vi "lcr tune mod.vi"() -> ()   [LabVIEW 2018]
uses:
  <vilib>/Analysis/NI_AALBase.lvlib
  <vilib>/Analysis/NI_AAL_SigProc.lvlib
  a6659894-6288-4190-a3c4-d24321de4737.vi
  <vilib>/DAQmx/write.llb/DAQmx Write (Analog DBL 1Chan 1Samp).vi
  <vilib>/DAQmx/create/channels.llb/DAQmx Create Channel (AO-Voltage-Basic).vi
  <vilib>/DAQmx/create/channels.llb/DAQmx Create Channel (AI-Voltage-Basic).vi
  2a3dda8a-b8aa-4613-8376-8d8c81e86704.vi
  <vilib>/Analysis/baseanly.llb/Mean (DBL).vi
  <vilib>/DAQmx/read.llb/DAQmx Read (Analog DBL 1Chan 1Samp).vi
panel:
  in  "stop":bool
  out "XY Graph 2":cluster{dbl[], dbl[]}(graph)={[0.0, 0.04950495049504951, 0.09900990099009901, 0.14851485148514854, 0.19801980198019803, 0.24752475247524752, 0.29702970297029707, 0.34653465346534656, 0.39603960396039606, 0.44554455445544555, 0.49504950495049505, 0.5445544554455446, 0.5940594059405941, 0.6435643564356436, 0.6930693069306931, 0.7425742574257426, 0.7920792079207921, 0.8415841584158417, 0.8910891089108911, 0.9405940594059407, 0.9900990099009901, 1.0396039603960396, 1.0891089108910892, 1.1386138613861387, 1.1881188118811883, 1.2376237623762376, 1.2871287128712872, 1.3366336633663367, 1.3861386138613863, 1.4356435643564358, 1.4851485148514851, 1.5346534653465347, 1.5841584158415842, 1.6336633663366338, 1.6831683168316833, 1.7326732673267327, 1.7821782178217822, 1.8316831683168318, 1.8811881188118813, 1.9306930693069309, 1.9801980198019802, 2.0297029702970297, 2.0792079207920793, 2.128712871287129, 2.1782178217821784, 2.227722772277228, 2.2772277227722775, 2.326732673267327, 2.3762376237623766, 2.4257425742574257, 2.4752475247524752, 2.5247524752475248, 2.5742574257425743, 2.623762376237624, 2.6732673267326734, 2.722772277227723, 2.7722772277227725, 2.821782178217822, 2.8712871287128716, 2.9207920792079207, 2.9702970297029703, 3.01980198019802, 3.0693069306930694, 3.118811881188119, 3.1683168316831685, 3.217821782178218, 3.2673267326732676, 3.316831683168317, 3.3663366336633667, 3.415841584158416, 3.4653465346534653, 3.514851485148515, 3.5643564356435644, 3.613861386138614, 3.6633663366336635, 3.712871287128713, 3.7623762376237626, 3.811881188118812, 3.8613861386138617, 3.9108910891089113, 3.9603960396039604, 4.00990099009901, 4.0594059405940595, 4.108910891089109, 4.158415841584159, 4.207920792079208, 4.257425742574258, 4.306930693069307, 4.356435643564357, 4.405940594059406, 4.455445544554456, 4.504950495049505, 4.554455445544555, 4.6039603960396045, 4.653465346534654, 4.702970297029704, 4.752475247524753, 4.801980198019802, 4.851485148514851, 4.900990099009901, 4.9504950495049505, 5.0], [3.6269698987299557, 3.6364573449364106, 3.6329899671345474, 3.6282543529705342, 3.629159309363951, 3.6287473758170243, 3.6300350736155056, 3.629924792216151, 3.6336451685832807, 3.63122870790565, 3.6250464609928272, 3.6300902143756275, 3.637209853485964, 3.6333467600149016, 3.630025342964688, 3.6329121214483715, 3.6278326887176044, 3.6270445008971244, 3.6230613953263267, 3.630712980049897, 3.6313000664504536, 3.6289971308177837, 3.6302329315360238, 3.6329153650017383, 3.6294609615211413, 3.63600000136827, 3.627411024462163, 3.6284100444363565, 3.6275861772915365, 3.6304729557761015, 3.629473935783759, 3.63204933151817, 3.6254162280427176, 3.627398050221512, 3.6295193457817647, 3.6331878249951624, 3.6319941907248854, 3.6278034965744808, 3.6220396703232898, 3.6262952359408596, 3.6273688580229018, 3.6348777256768994, 3.6264476837299795, 3.633719770708133, 3.6360843342001994, 3.6295290764943395, 3.6302459057692227, 3.6275504979969018, 3.6291366044222984, 3.632672097159256, 3.6235057645788302, 3.6296361143819986, 3.6328342757014656, 3.6316990257371065, 3.62449829739106, 3.629097681502316, 3.624031223133673, 3.6252702673373305, 3.6278229579737187, 3.6336192199758655, 3.6273623709287937, 3.621828838189813, 3.631844986473933, 3.625150255217819, 3.625172960190463, 3.6291917451084803, 3.6294479872235597, 3.619243711878944, 3.6345630992469626, 3.6295615122275064, 3.6293896029595634, 3.6309984143274994, 3.6328083271841956, 3.6245664123692127, 3.6280954180164486, 3.627754843002688, 3.6386662170654303, 3.62156935249656, 3.6349231357495135, 3.637310404233228, 3.6250724094892646, 3.6337684242639474, 3.638114809914663, 3.625224857360931, 3.6308427229410554, 3.637796939897928, 3.6351177500173657, 3.6332105299869375, 3.632360714266952, 3.635607529201048, 3.6308200179121477, 3.634835559237383, 3.6350820706466345, 3.6253027030898712, 3.633823564980328, 3.623252765981493, 3.6300156121881697, 3.6215855703379147, 3.6359124249670454, 3.630398353613972, 3.6265287730372937, 3.6269212451486847]}
  in  "width":i32=3 min=3
  in  "threshold":dbl format="%0.2f"
  in  "sample length":i32=100
  in  "Step length (ms)":dbl
  in  "step size":dbl
  out "estimated polarization":dbl
  in  "background intensity":dbl
  in  "polarimeter angle":dbl
  in  "pressure factor":dbl
  out "min location":dbl
  out "min value":dbl
  out "max location":dbl
  out "max value":dbl
  out "average":dbl
  in  "laser tune voltage":dbl=3.79 min=0.0 max=4.0 step=0.01
  out "max value":dbl=3.6386662170654303
  out "min value":dbl=3.619243711878944
  out "Voltage at min":dbl=3.316831683168317
  out "Voltage at max":dbl=3.7623762376237626
  out "Current Voltage":dbl=5.0
  out "XY Graph":cluster{dbl[], dbl[]}(graph)={[0.0, 0.04950495049504951, 0.09900990099009901, 0.14851485148514854, 0.19801980198019803, 0.24752475247524752, 0.29702970297029707, 0.34653465346534656, 0.39603960396039606, 0.44554455445544555, 0.49504950495049505, 0.5445544554455446, 0.5940594059405941, 0.6435643564356436, 0.6930693069306931, 0.7425742574257426, 0.7920792079207921, 0.8415841584158417, 0.8910891089108911, 0.9405940594059407, 0.9900990099009901, 1.0396039603960396, 1.0891089108910892, 1.1386138613861387, 1.1881188118811883, 1.2376237623762376, 1.2871287128712872, 1.3366336633663367, 1.3861386138613863, 1.4356435643564358, 1.4851485148514851, 1.5346534653465347, 1.5841584158415842, 1.6336633663366338, 1.6831683168316833, 1.7326732673267327, 1.7821782178217822, 1.8316831683168318, 1.8811881188118813, 1.9306930693069309, 1.9801980198019802, 2.0297029702970297, 2.0792079207920793, 2.128712871287129, 2.1782178217821784, 2.227722772277228, 2.2772277227722775, 2.326732673267327, 2.3762376237623766, 2.4257425742574257, 2.4752475247524752, 2.5247524752475248, 2.5742574257425743, 2.623762376237624, 2.6732673267326734, 2.722772277227723, 2.7722772277227725, 2.821782178217822, 2.8712871287128716, 2.9207920792079207, 2.9702970297029703, 3.01980198019802, 3.0693069306930694, 3.118811881188119, 3.1683168316831685, 3.217821782178218, 3.2673267326732676, 3.316831683168317, 3.3663366336633667, 3.415841584158416, 3.4653465346534653, 3.514851485148515, 3.5643564356435644, 3.613861386138614, 3.6633663366336635, 3.712871287128713, 3.7623762376237626, 3.811881188118812, 3.8613861386138617, 3.9108910891089113, 3.9603960396039604, 4.00990099009901, 4.0594059405940595, 4.108910891089109, 4.158415841584159, 4.207920792079208, 4.257425742574258, 4.306930693069307, 4.356435643564357, 4.405940594059406, 4.455445544554456, 4.504950495049505, 4.554455445544555, 4.6039603960396045, 4.653465346534654, 4.702970297029704, 4.752475247524753, 4.801980198019802, 4.851485148514851, 4.900990099009901, 4.9504950495049505, 5.0], [3.6269698987299557, 3.6364573449364106, 3.6329899671345474, 3.6282543529705342, 3.629159309363951, 3.6287473758170243, 3.6300350736155056, 3.629924792216151, 3.6336451685832807, 3.63122870790565, 3.6250464609928272, 3.6300902143756275, 3.637209853485964, 3.6333467600149016, 3.630025342964688, 3.6329121214483715, 3.6278326887176044, 3.6270445008971244, 3.6230613953263267, 3.630712980049897, 3.6313000664504536, 3.6289971308177837, 3.6302329315360238, 3.6329153650017383, 3.6294609615211413, 3.63600000136827, 3.627411024462163, 3.6284100444363565, 3.6275861772915365, 3.6304729557761015, 3.629473935783759, 3.63204933151817, 3.6254162280427176, 3.627398050221512, 3.6295193457817647, 3.6331878249951624, 3.6319941907248854, 3.6278034965744808, 3.6220396703232898, 3.6262952359408596, 3.6273688580229018, 3.6348777256768994, 3.6264476837299795, 3.633719770708133, 3.6360843342001994, 3.6295290764943395, 3.6302459057692227, 3.6275504979969018, 3.6291366044222984, 3.632672097159256, 3.6235057645788302, 3.6296361143819986, 3.6328342757014656, 3.6316990257371065, 3.62449829739106, 3.629097681502316, 3.624031223133673, 3.6252702673373305, 3.6278229579737187, 3.6336192199758655, 3.6273623709287937, 3.621828838189813, 3.631844986473933, 3.625150255217819, 3.625172960190463, 3.6291917451084803, 3.6294479872235597, 3.619243711878944, 3.6345630992469626, 3.6295615122275064, 3.6293896029595634, 3.6309984143274994, 3.6328083271841956, 3.6245664123692127, 3.6280954180164486, 3.627754843002688, 3.6386662170654303, 3.62156935249656, 3.6349231357495135, 3.637310404233228, 3.6250724094892646, 3.6337684242639474, 3.638114809914663, 3.625224857360931, 3.6308427229410554, 3.637796939897928, 3.6351177500173657, 3.6332105299869375, 3.632360714266952, 3.635607529201048, 3.6308200179121477, 3.634835559237383, 3.6350820706466345, 3.6253027030898712, 3.633823564980328, 3.623252765981493, 3.6300156121881697, 3.6215855703379147, 3.6359124249670454, 3.630398353613972, 3.6265287730372937, 3.6269212451486847]}
  in  "End Voltage":dbl=5.0 min=0.0 max=25.0 step=0.001 format="%#.3f"
  in  "VISA resource name":refnum<visa-resource-name>="LCC25"
  in  "Start Voltage":dbl min=0.0 max=25.0 step=0.001 format="%#.3f"
  # "This VI sweeps the LCR driving voltage.   LCR slow axis should be aligned to roughly 45 degrees from the \ntransmission axis of the linear plarizer.  The max and min of graph represent citical values such as 1/4 wave,\n3/4 wave, etc.  The corresponding Voltages are then used fine tune the alignemnt and to make polarization\nmeasurements."
  # "X"
  # "Y"
  # "(ignore for background measurements)"
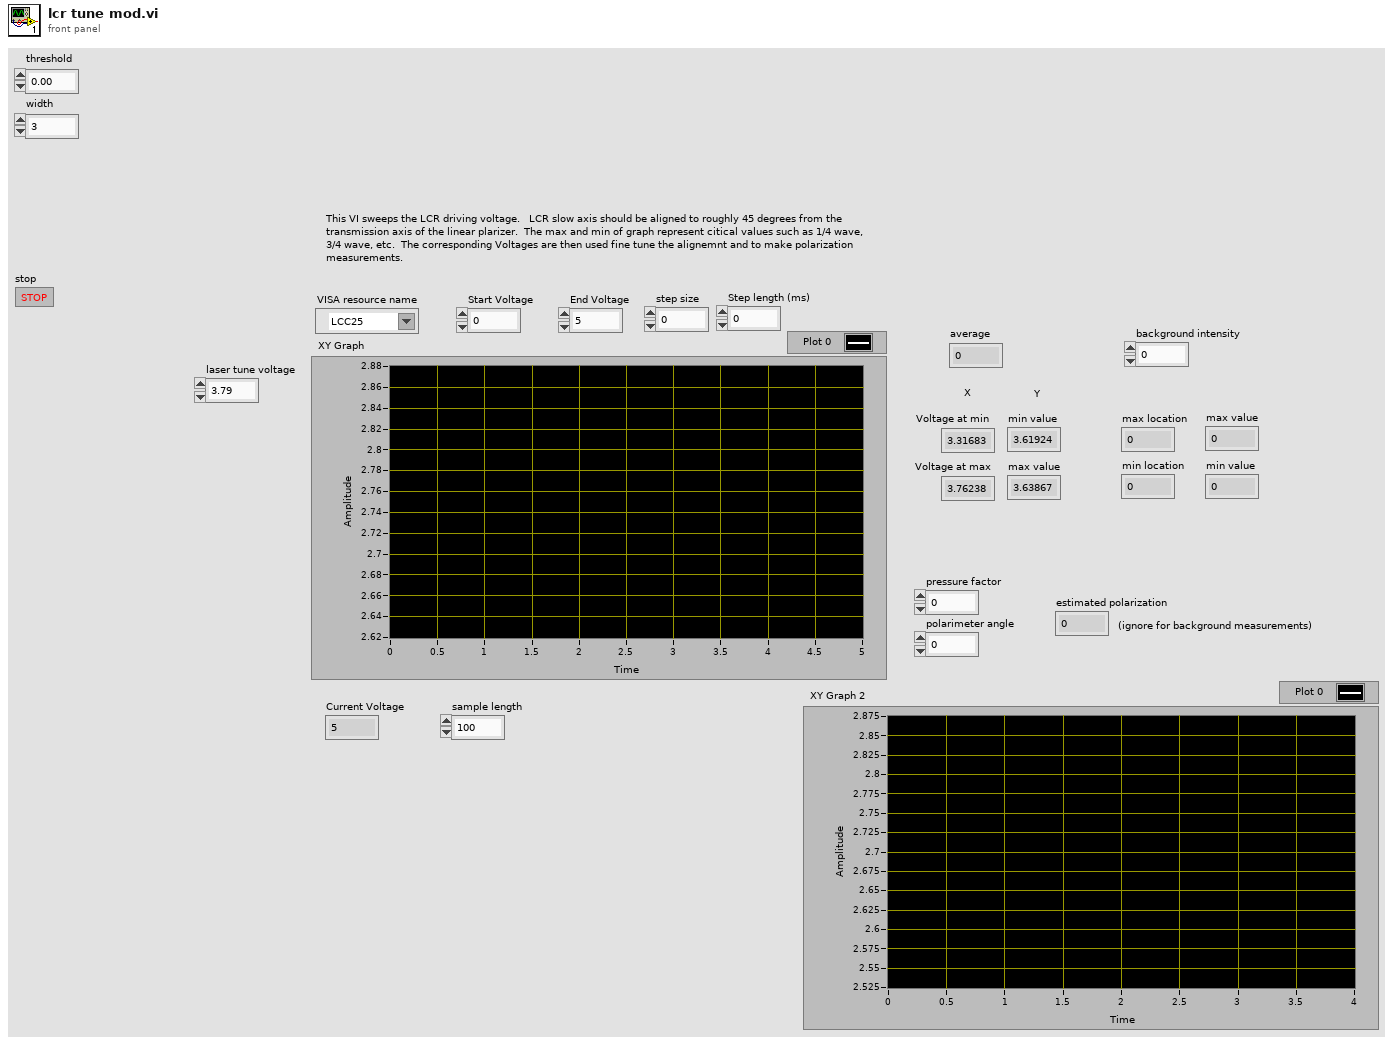
[diagram p1: front panel]
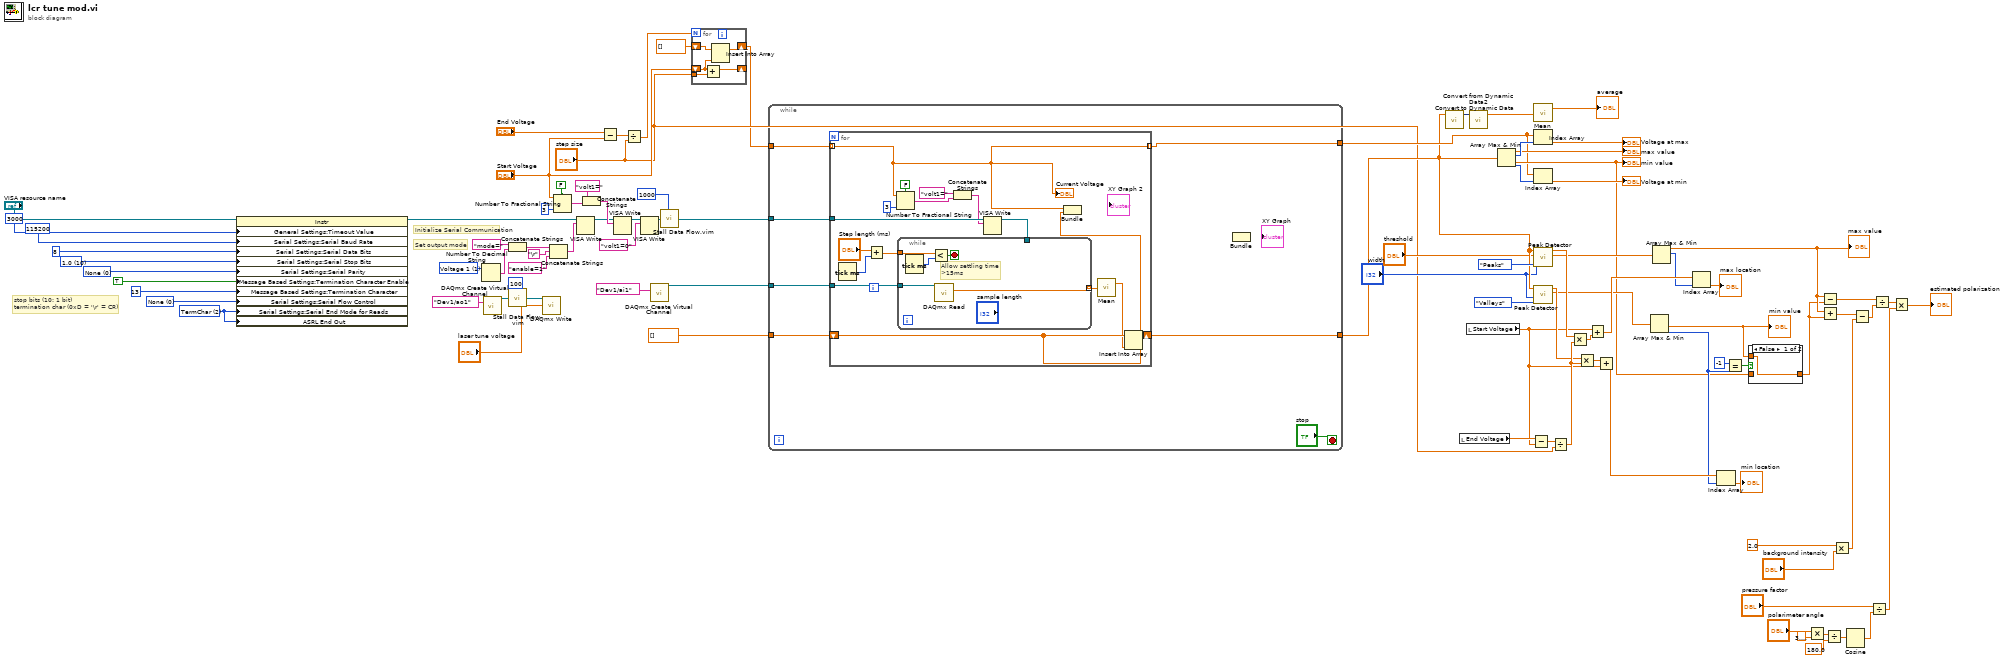
[diagram p0: block diagram]
diagram:
  w88 = u16 1 items=["Modulate", "Voltage 1", "Voltage 2"] ("Output Mode")
  w89 = u16 2 items=["None", "LastBit", "TermChar"] ("Serial Settings:Serial End Mode for Reads")
  w93 = u16 0 items=["None", "XON/XOFF", "RTS/CTS", "XON/XOFF & RTS/CTS", "DTR/DSR", "XON/XOFF & DTR/DSR"] ("flow control (0:none)")
  w91 = u16 0 items=["None", "Odd", "Even", "Mark", "Space"] ("Serial Settings:Parity")
  w95 = u16 10 items=["1.0"=10, "1.5"=15, "2.0"=20]
  # "stop bits (10: 1 bit)\ntermination char (0xD = '\\r' = CR)"
  # "Set output mode"
  # "Initialize Serial Communication"
  n1 = property class="Instr"(reference="VISA resource name", "General Settings:Timeout Value"=u32 3000 ("timeout (10sec)"), "Serial Settings:Serial Baud Rate"=u32 115200 ("baud rate (9600)115200"), "Serial Settings:Serial Data Bits"=u16 8 ("data bits (8)"), "Serial Settings:Serial Stop Bits"=w95, "Serial Settings:Serial Parity"=w91, "Message Based Settings:Termination Character Enable"=TRUE ("Enable Termination\nChar (T)"), "Message Based Settings:Termination Character"=u8 13, "Serial Settings:Serial Flow Control"=w93, "Serial Settings:Serial End Mode for Reads"=w89, "ASRL End Out"=w89) -> (reference out=w73:refnum<visa-resource-name>)  [unwired: 1 in, 1 out]
  n2 = Number To Decimal String(number=w88) -> (decimal integer string=w87:string)  [unwired: 1 in]
  n3 = call-poly <vilib>:"DAQmx Create Virtual Channel.vi"("physical channels"=tag "Dev1/ao1") -> ("task out"=w64:refnum<k21>)  [unwired: 13 in, 1 out]
  n4 = Concatenate Strings("mode=" ("string"), w87) -> (w75:string)
  n5 = call "Stall Data Flow.vim"("value in"=w64, "milliseconds to wait"=u32 100) -> ("value out"=w15:refnum<k21>)  [unwired: 1 out]
  n6 = call-poly <vilib>:"DAQmx Write.vi"("task/channels in"=w15, "data"="laser tune voltage") -> ()  [unwired: 11 in, 3 out]
  n7 = Concatenate Strings(w75, "\r", "enable=1" ("write buffer")) -> (w74:string)
  n8 = Number To Fractional String(use system decimal point (T)=FALSE, number="Start Voltage", precision (6)=i16 3) -> (F-format string=w69:string)  [unwired: 1 in]
  n9 = VISA Write(VISA resource name=w73, write buffer=w74) -> (VISA resource name out=w66:refnum<visa-resource-name>)  [unwired: 1 in, 2 out]
  n10 = Concatenate Strings("volt1=" ("string"), w69) -> (w67:string)
  n11 = Subtract(x="End Voltage", y="Start Voltage") -> (x-y=w84:dbl)
  n12 = VISA Write(VISA resource name=w66, write buffer=w67) -> (VISA resource name out=w29:refnum<visa-resource-name>)  [unwired: 1 in, 2 out]
  n13 = Divide(x=w84, y="step size") -> (x/y=w5:dbl)
  n14 = VISA Write(VISA resource name=w29, write buffer="volt1=0" ("string")) -> (VISA resource name out=w53:refnum<visa-resource-name>)  [unwired: 1 in, 2 out]
  n15 = call-poly <vilib>:"DAQmx Create Virtual Channel.vi"("physical channels"=tag "Dev1/ai1") -> ("task out"=w13:refnum<k21>)  [unwired: 13 in, 1 out]
  n16 = call "Stall Data Flow.vim"("value in"=w53, "milliseconds to wait"=u32 1000) -> ("value out"=w7:refnum<visa-resource-name>)  [unwired: 1 out]
  n17 = for {
    N: w5 -> [_]
    shift-right: [w100] -> w1
    shift-left: dbl[] [] -> [w101]
    tunnel: "step size" -> [w99]
    shift-right: [w98] -> _
    shift-left: "Start Voltage" -> [w97]
    n18 = Add(x=w97, y=w99) -> (x+y=w98:dbl)
    n19 = Insert Into Array(array=w101, new element=w97) -> (w100:dbl[])  [unwired: 1 in]
  }
  n20 = while {
    tunnel: [w108] -> w16
    tunnel: w13 -> [w107]
    tunnel: [w106] -> w11
    tunnel: dbl[] [] -> [w105]
    tunnel: w1 -> [w104]
    tunnel: w7 -> [w103]
    stop <- "stop" stop-if-true
    n21 = for {
      tunnel: w103 -> [w120]
      tunnel: w107 -> [w118]
      shift-right: [w113] -> w106
      shift-left: w105 -> [w112]
      tunnel: w104 -> [w109] mode=indexing
      tunnel: [w109] -> w108 mode=indexing
      n22 = Tick Count (ms)() -> (millisecond timer value=w117:u32)
      n23 = Add(x="Step length (ms)", y=w117) -> (x+y=w115:dbl)
      n24 = Number To Fractional String(use system decimal point (T)=FALSE, number=w109, precision (6)=i16 3) -> (F-format string=w122:string)  [unwired: 1 in]
      n25 = Concatenate Strings("volt1=" ("string"), w122) -> (w119:string)
      n26 = VISA Write(VISA resource name=w120, write buffer=w119) -> (VISA resource name out=w114:refnum<visa-resource-name>)  [unwired: 1 in, 2 out]
      n27 = while {
        tunnel: w118 -> [w129]
        tunnel: w115 -> [w128]
        tunnel: w114 -> [_]
        tunnel: [w125] -> w111 mode=indexing
        stop <- w126 stop-if-true
        # "Allow settling time\n>15ms"
        n28 = Tick Count (ms)() -> (millisecond timer value=w127:u32)
        n29 = Less?(x=w128, y=w127) -> (x < y?=w126:bool)
        n30 = call-poly <vilib>:"DAQmx Read.vi"("task/channels in"=w129) -> ("data"=w125:dbl)  [unwired: 12 in, 2 out]
      }
      n31 = Bundle(w109, w112) -> ()  [unwired: 1 in, 1 out]
      n32 = call-poly <vilib>:"Mean.vi"("X"=w111) -> ("mean"=w110:dbl)  [unwired: 1 out]
      n33 = Insert Into Array(array=w112, new element=w110) -> (w113:dbl[])  [unwired: 1 in]
      "Current Voltage" <- w109
    }
    n34 = Bundle() -> ()  [unwired: 3 in, 1 out]
  }
  n35 = call "Convert to Dynamic Data"("Array"=w11) -> ("Dynamic Data Type"=w27:dynamicdata)  [unwired: 3 in]
  n36 = local read "End Voltage"() -> (w62:dbl)
  n37 = local read "Start Voltage"() -> (w44:dbl)
  n38 = call "Convert from Dynamic Data2"("Dynamic Data Type"=w27) -> ("Array"=w52:dbl[])  [unwired: 3 in]
  n39 = Array Max & Min(array=w11) -> (max value=→"max value":dbl, max index (indices)=w81:i32, min value=w20:dbl, min index (indices)=w82:i32)
  "min value" <- w20
  n40 = Subtract(x=w62, y=w44) -> (x-y=w55:dbl)
  n41 = call-poly <vilib>:"Mean.vi"("X"=w52) -> ("mean"=→"average":dbl)  [unwired: 1 out]
  n42 = Index Array(array=w16, index=w81) -> (element=→"Voltage at max":dbl)
  n43 = Index Array(array=w16, index=w82) -> (element=→"Voltage at min":dbl)
  n44 = call <vilib>:"Peak Detector.vi"("peaks/valleys"=enum32{"Peaks", "Valleys"}."Peaks", "width"="width", "threshold"="threshold", "X"=w11) -> ("Amplitudes"=w51:dbl[], "Locations"=w61:dbl[])  [unwired: 3 in, 3 out]
  n45 = call <vilib>:"Peak Detector.vi"("peaks/valleys"=enum32{"Peaks", "Valleys"}."Valleys", "width"="width", "X"=w11) -> ("Amplitudes"=w47:dbl[], "Locations"=w57:dbl[])  [unwired: 4 in, 3 out]
  n46 = Divide(x=w55, y="step size") -> (x/y=w58:dbl)
  n47 = Multiply(x=w61, y=w58) -> (x*y=w60:dbl[])
  n48 = Multiply(x=w57, y=w58) -> (x*y=w56:dbl[])
  n49 = Add(x=w44, y=w60) -> (x+y=w50:dbl[])
  n50 = Add(x=w56, y=w44) -> (x+y=w46:dbl[])
  n51 = Array Max & Min(array=w47) -> (min value=w19:dbl, min index (indices)=w23:i32)  [unwired: 2 out]
  "min value" <- w19
  n52 = Array Max & Min(array=w51) -> (max value=w36:dbl, max index (indices)=w49:i32)  [unwired: 2 out]
  "max value" <- w36
  n53 = Index Array(array=w50, index=w49) -> (element=→"max location":dbl)
  n54 = Index Array(array=w46, index=w23) -> (element=→"min location":dbl)
  n55 = Equal?(x=-1, y=w23) -> (x = y?=w21:bool)
  n56 = case shown="False" w21 {
    tunnel: w19 -> [w130 _]
    tunnel: w20 -> [_ w131]
    tunnel: [w130 w131] -> w18
    frame False {
    }
    frame True {
    }
  }
  n57 = Multiply(x="polarimeter angle", y=3.141592653589793) -> (x*y=w41:dbl)
  n58 = Subtract(x=w36, y=w18) -> (x-y=w25:dbl)
  n59 = Add(x=w36, y=w18) -> (x+y=w35:dbl)
  n60 = Divide(x=w41, y=180.0) -> (x/y=w39:dbl)
  n61 = Multiply(x=2.0, y="background intensity") -> (x*y=w33:dbl)
  n62 = Cosine(x=w39) -> (cos(x)=w37:dbl)
  n63 = Subtract(x=w35, y=w33) -> (x-y=w32:dbl)
  n64 = Divide(x="pressure factor", y=w37) -> (x/y=w24:dbl)
  n65 = Divide(x=w25, y=w32) -> (x/y=w31:dbl)
  n66 = Multiply(x=w31, y=w24) -> (x*y=→"estimated polarization":dbl)
